vi "Configure Services.vi"(8 "error in (no error)":errorcluster, 11 "WS Test Server in":refnum<class "WS Test Server Subscriber.lvclass">) -> (0 "error out":errorcluster, 3 "WS Test Server out":refnum<class "WS Test Server Subscriber.lvclass">)   [LabVIEW 2021, in "Secure Echo Broadcast Test Server Manager.lvlib" / "WS Test Server Subscriber.lvclass"]
uses:
  WS Test Server Subscriber.lvclass
  C:/Program Files/National Instruments/LabVIEW 2021/vi.lib/ActorFramework/Actor/Actor.lvclass
  WS Test Server Subscriber Messages/WebSocket Service Enqueuer Msg/WebSocket Service Enqueuer Msg.lvclass
  C:/Projects/WebSocket-Actor/WebSocket Actor/Abstract Messages/WebSocket Server-Service Enqueuer Msg/WebSocket Server-Service Enqueuer Msg.lvclass
  WS Test Server Subscriber Messages/Server Connection Handler Msg/Server Connection Handler Msg.lvclass
  C:/Projects/WebSocket-Actor/WebSocket Actor/Abstract Messages/WebSocket Connection Handler Msg/WebSocket Connection Handler Msg.lvclass
  <vilib>/ActorFramework/Actor/Actor.lvclass/Actor.ctl
  <vilib>/ActorFramework/Message Enqueuer/Message Enqueuer.lvclass/Message Enqueuer.ctl
  WS Test Server Subscriber.lvclass/WS Test Server Subscriber.ctl
  <vilib>/ActorFramework/Message Enqueuer/Init from Existing Queue.vi
  <vilib>/ActorFramework/Message Enqueuer/Message Enqueuer.lvclass
  WebSocket Actor/WebSocket Server Messages/Add Service Msg/Add Service Msg.lvclass
  <vilib>/ActorFramework/Actor/Actor.lvclass
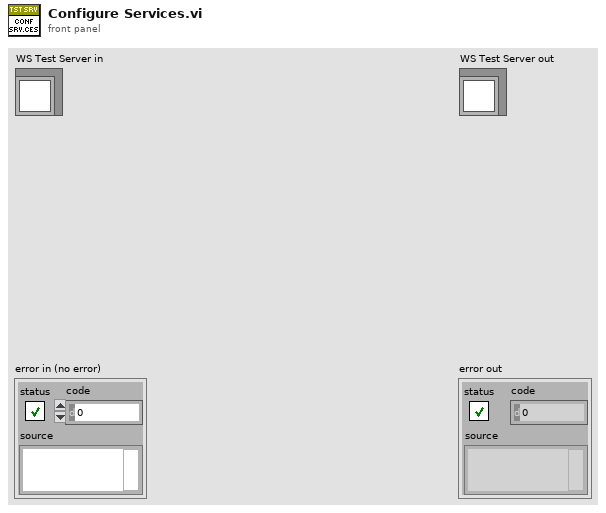
[diagram p1: front panel]
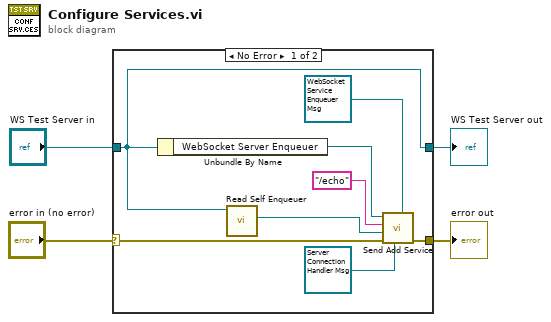
[diagram p0: block diagram]
diagram:
  n1 = case shown="No Error" "error in (no error)" {
    selector: "error in (no error)" -> [w9 w14]
    tunnel: [w8 w14] -> w3
    tunnel: [w6 w13] -> w1
    tunnel: "WS Test Server in" -> [w6 w13]
    frame No Error {
      n2 = Unbundle By Name(w6) -> ("WebSocket Server Enqueuer"=w11:refnum<class "Message Enqueuer.lvclass">)
      n3 = call <vilib>:"Read Self Enqueuer.vi"("Actor"=w6) -> ("Self Enqueuer"=w5:refnum<class "Message Enqueuer.lvclass">)  [unwired: 10 in]
      n4 = call "Send Add Service.vi"("Receive Connection Enqueuer Handler"=refnum<class "WebSocket Service Enqueuer Msg.lvclass"> refnum ("Echo Broadcast Test With Server Manager.lvlib:WebSocket Service Enqueuer Msg.lvclass"), "WebSocket Data Handler"=refnum<class "Server Connection Handler Msg.lvclass"> refnum ("Echo Broadcast Test With Server Manager.lvlib:Server Connection Handler Msg.lvclass"), "error in (no error)"=w9, "Subscriber Enqueuer"=w5, "Service Name"="/echo", "Message Enqueuer in"=w11) -> ("error out"=w8:errorcluster)  [unwired: 4 in, 1 out]
    }
    frame Error {
    }
  }
  "error out" <- w3
  "WS Test Server out" <- w1
